vi "automated_Strain_attempt.vi"() -> ()   [LabVIEW 2014]
uses:
  <vilib>/vision/NI_Vision_Development_Module.lvlib
  <instrlib>/KD Scientific 2XX Series/KD Scientific 2XX Series.lvlib
panel:
  out "Diameter Selection":T1(plugin-control)
  out "di2":dbl
  out "di1":dbl
  out "d1":dbl
  out "d2":dbl
  out "Distances":dbl[](array[numeric])
  out "S2":dbl
  out "S1":dbl
  in  "Number of Cycles":i32
  in  "Min Pressure":dbl
  in  "Max Pressure":dbl
  out "Status":T2
  in  "stop 2":bool
  out "Delivered Volume":dbl
  out "Units":string
  in  "Baud Rate (9600)":u32(ring)=9600 items=["300"=300, "1200"=1200, "2400"=2400, "4800"=4800, "9600"=9600]
  in  "Withdrawal Settings":T3={"Flow Rate (5)"=5.0, "Volume (10)"=10.0, "Volume Units (ml)"=enum."milliliters (ml)", "Rate Units (ml/min.)"=enum."milliliters per minute (ml/min.)"} {"Volume (10)" format="%#.3g"}
  in  "Diameter (8.75 mm)":dbl=8.75
  in  "Infusion Settings":T3={"Flow Rate (5)"=5.0, "Volume (10)"=10.0, "Volume Units (ml)"=enum."milliliters (ml)", "Rate Units (ml/min.)"=enum."milliliters per minute (ml/min.)"}
  in  "Address (0)":i32 format="%0.0f"
  in  "error in (no error)":errorcluster
  in  "VISA resource name":refnum<visa-resource-name>="COM1"
  in  "stop 4":bool
  in  "stop":bool
  out "Strain Selection":T1(plugin-control)
  out "Particle Measurements (Pixels) (Particle Analysis 1)":dbl[][](array[numeric]) format="%.2f"
  out "subarray":dbl[](array[numeric])
  out "The diameter":dbl[](array[numeric])
  in  "stop (F)":bool
  out "Data from Transducer":dynamicdata(graph) caption="Voltage from Transducer V"
  out "Voltage from pressure transducer":dbl[](array[numeric])
  out "Pressure mm Hg":dbl[](graph)
  in  "Calibration factor":dbl[](array[numeric])
  in  "Zero Error":dbl[](array[numeric])
  out "pressure mm Hg":dbl[](array[numeric])
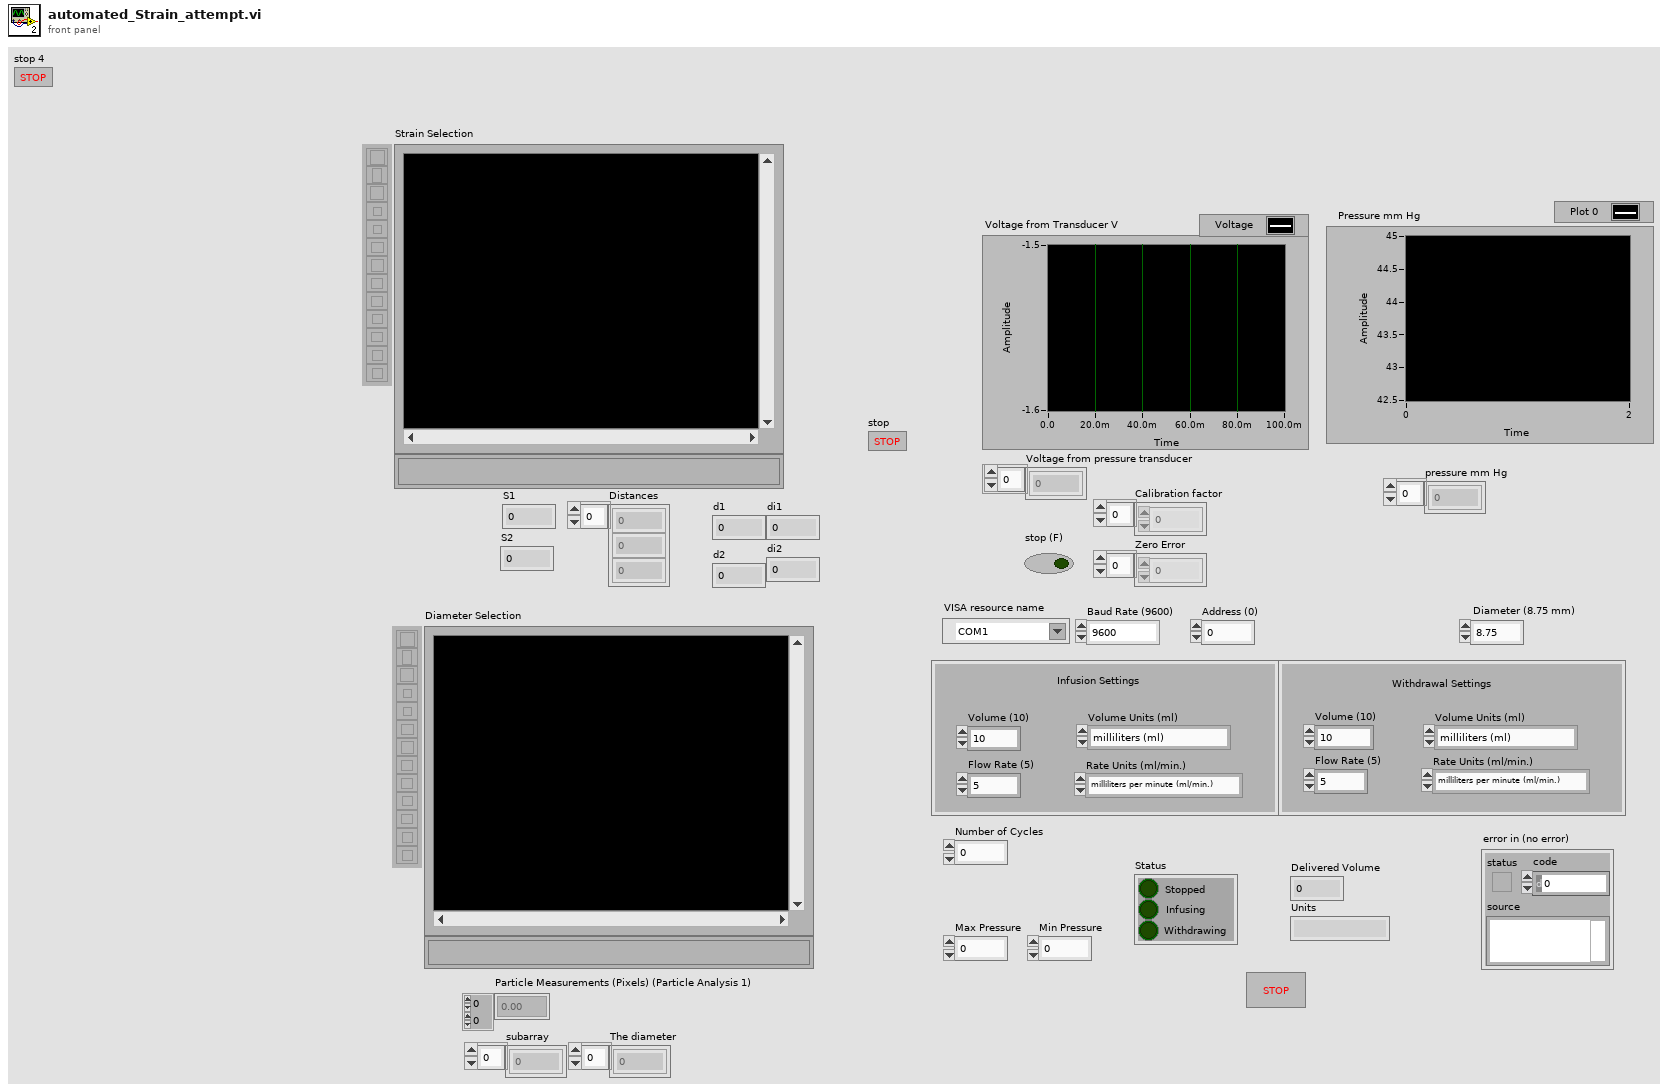
[diagram p1: front panel]
types:
  T1 = typedef "IMAQ Image.ctl" = refnum<image>
  T2 = cluster{"Stopped":bool, "Infusing":bool, "Withdrawing":bool}
  T3 = cluster{"Flow Rate (5)":dbl, "Volume (10)":dbl, "Volume Units (ml)":enum16{"milliliters (ml)", "microliters (ul)"}, "Rate Units (ml/min.)":enum16{"milliliters per minute (ml/min.)", "milliliters per hour (ml/hr.)", "microliters per minute (ul/min.)", "microliters per hour (ul/hr.)"}}
  T4 = typedef "Board Id" = u8
  T5 = typedef "ROI Descriptor" = cluster{"Global Rectangle":i32[], "Contours":cluster{"ID":enum32{"External", "Internal"}, "Type":u32, "Coordinates":i32[]}[]}
  T6 = enum16{"milliliters per minute (ml/min.)", "milliliters per hour (ml/hr.)", "microliters per minute (ul/min.)", "microliters per hour (ul/hr.)"}
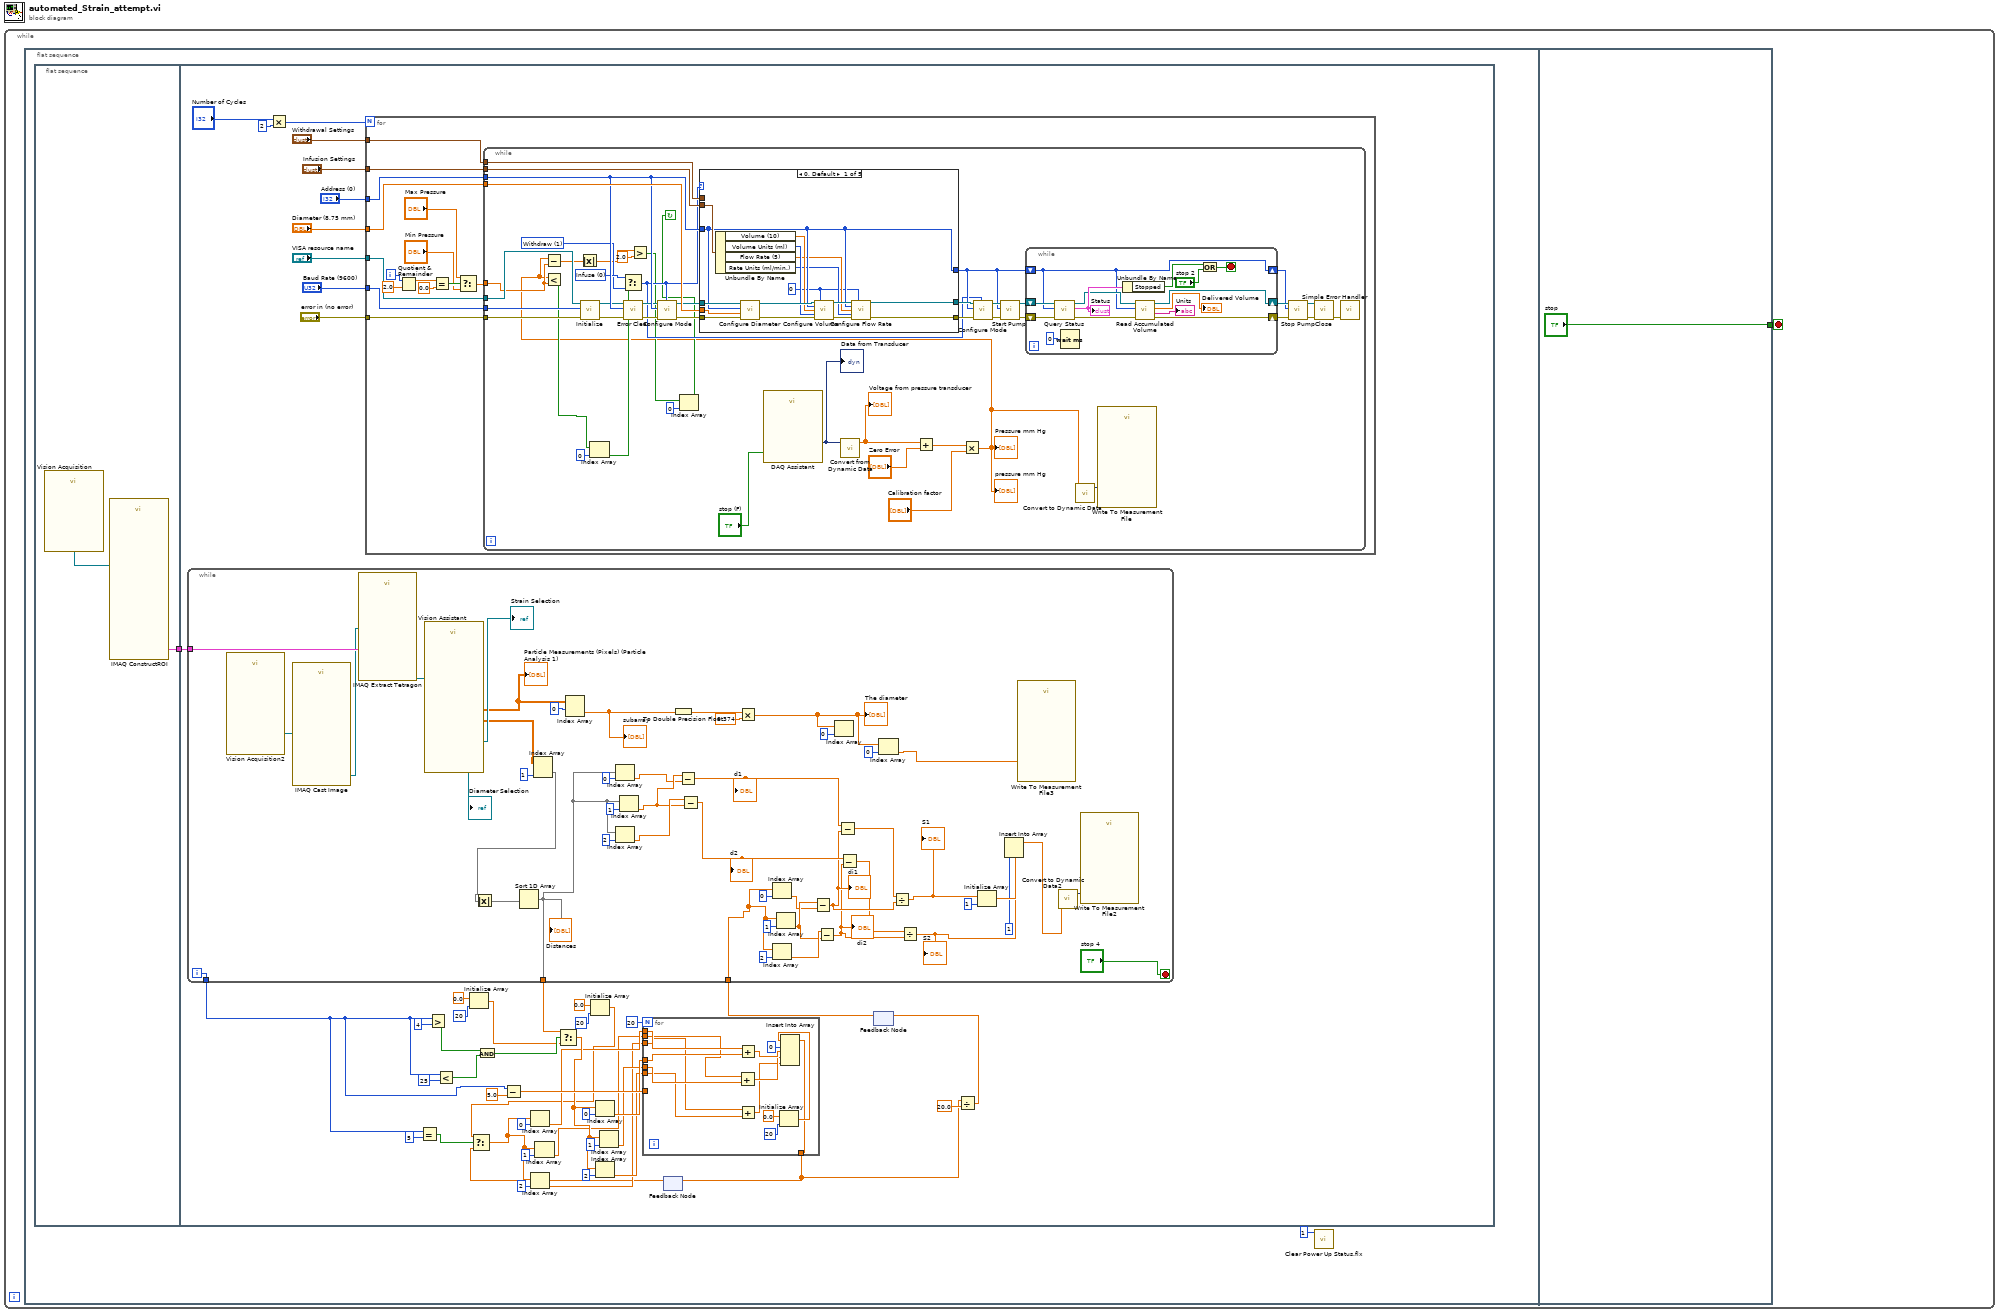
[diagram p0: block diagram]
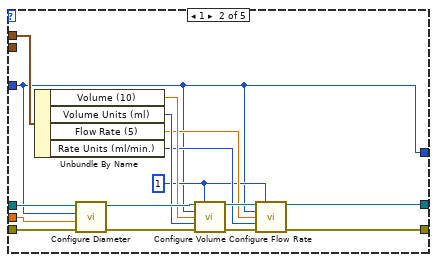
[diagram p2: hidden frame]
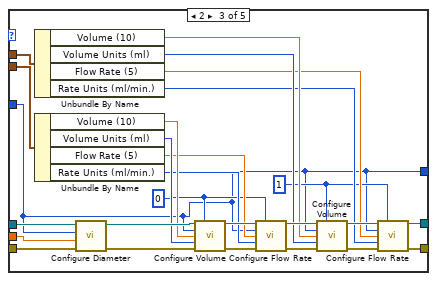
[diagram p3: hidden frame]
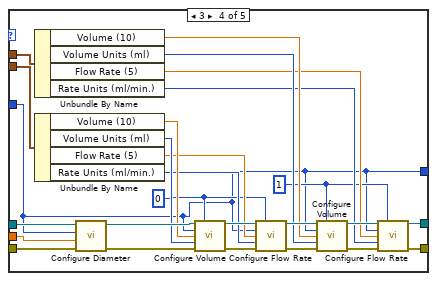
[diagram p4: hidden frame]
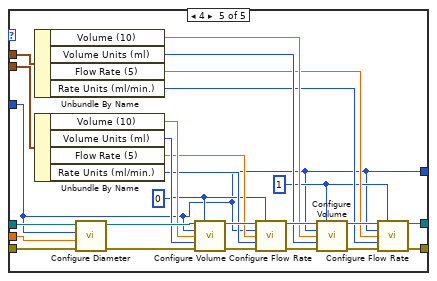
[diagram p5: hidden frame]
diagram:
  n1 = while {
    stop <- w1 stop-if-true
    n2 = flat-sequence {
      tunnel: ["stop"] -> w1
      frame #0 {
        n3 = flat-sequence {
          tunnel: [w4] -> w3
          tunnel: w3 -> [w53]
          frame #0 {
            n4 = call "Vision Acquisition"() -> ("Image Out"=w5:T1)  [unwired: 26 in, 1 out]
            n5 = call "IMAQ ConstructROI"("Image"=w5) -> ("ROI Descriptor Out"=w4:T5)  [unwired: 7 in, 3 out]
          }
          frame #1 {
            n6 = Multiply(x="Number of Cycles", y=2) -> (x*y=w52:i32)
            n7 = for {
              N: w52 -> [_]
              tunnel: "VISA resource name" -> [w82]
              tunnel: "error in (no error)" -> [w81]
              tunnel: "Infusion Settings" -> [w80]
              tunnel: "Withdrawal Settings" -> [w79]
              tunnel: "Diameter (8.75 mm)" -> [w78]
              tunnel: "Baud Rate (9600)" -> [w77]
              tunnel: "Address (0)" -> [w76]
              i -> [w74]
              n8 = Quotient & Remainder(x=w74, y=2.0) -> (x-y*floor(x/y)=w72:dbl)  [unwired: 1 out]
              n9 = Equal?(x=w72, y=0.0) -> (x = y?=w71:bool)
              n10 = Select(t="Max Pressure", s=w71, f="Min Pressure") -> (s? t:f=w68:dbl)
              n11 = while {
                tunnel: w82 -> [w129]
                tunnel: w81 -> [w128]
                tunnel: w80 -> [w127]
                tunnel: w79 -> [w126]
                tunnel: w78 -> [w125]
                tunnel: w77 -> [w124]
                tunnel: w76 -> [w123]
                tunnel: w68 -> [w100]
                stop <- w85 continue-if-true
                w102 = u16 1 items=["Withdraw"=1]
                w103 = u16 0 items=["Infuse"] ("Mode (infuse)")
                n12 = call <instrlib>:"Initialize.vi"("error in (no error)"=w128, "Baud Rate (9600)"=w124, "VISA resource name"=w129) -> ("error out"=w105:errorcluster, "VISA resource name out"=w104:refnum<visa-resource-name>)  [unwired: 7 in]
                n13 = call <instrlib>:"Error Clear.vi"("error in (no error)"=w105, "Address (0)"=w123, "VISA resource name"=w104) -> ("error out"=w106:errorcluster, "VISA resource name out"=w107:refnum<visa-resource-name>)  [unwired: 6 in, 1 out]
                n14 = call "DAQ Assistant"("stop (T)"="stop (F)") -> ("data"=w91:dynamicdata)  [unwired: 16 in, 2 out]
                "Data from Transducer" <- w91
                n15 = call "Convert from Dynamic Data"("Dynamic Data Type"=w91) -> ("Array"=w94:dbl[])  [unwired: 3 in]
                "Voltage from pressure transducer" <- w94
                n16 = Add(x=w94, y="Zero Error") -> (x+y=w92:dbl[])
                n17 = Multiply(x=w92, y="Calibration factor") -> (x*y=w84:dbl[])
                "Pressure mm Hg" <- w84
                "pressure mm Hg" <- w84
                n18 = Subtract(x=w84, y=w100) -> (x-y=w99:dbl[])
                n19 = Less?(x=w84, y=w100) -> (x < y?=w90:bool[])
                n20 = Absolute Value(x=w99) -> (abs(x)=w98:dbl[])
                n21 = Index Array(array=w90, index=0) -> (element=w88:bool)
                n22 = Select(t=w103, s=w88, f=w102) -> (s? t:f=w101:u16)
                n23 = Greater?(x=w98, y=2.0) -> (0:w87:bool[])
                n24 = call <instrlib>:"Configure Mode.vi"("Mode (infuse)"=w101, "error in (no error)"=w106, "Address (0)"=w123, "VISA resource name"=w107) -> ("error out"=w109:errorcluster, "VISA resource name out"=w108:refnum<visa-resource-name>)  [unwired: 6 in]
                n25 = Index Array(array=w87, index=0) -> (element=w85:bool)
                n26 = case shown="0, Default" w101 {
                  tunnel: w127 -> [w139 _ w187 w213 w239]
                  tunnel: w126 -> [_ w161 w186 w212 w238]
                  tunnel: w108 -> [w145 w160 w185 w211 w237]
                  tunnel: w109 -> [w144 w156 w184 w210 w236]
                  tunnel: w125 -> [w138 w152 w167 w193 w219]
                  tunnel: [w137 w146 w162 w188 w214] -> w110
                  tunnel: w123 -> [w137 w146 w162 w188 w214]
                  tunnel: [w132 w157 w164 w190 w216] -> w114
                  tunnel: [w131 w153 w163 w189 w215] -> w113
                  frame 0, Default {
                    w130 = 0
                    n27 = Unbundle By Name(w139) -> ("Volume (10)"=w136:dbl, "Volume Units (ml)"=w135:enum16{"milliliters (ml)", "microliters (ul)"}, "Flow Rate (5)"=w134:dbl, "Rate Units (ml/min.)"=w133:T6)
                    n28 = call <instrlib>:"Configure Diameter.vi"("error in (no error)"=w144, "Diameter (8.75 mm)"=w138, "Address (0)"=w137, "VISA resource name"=w145) -> ("error out"=w142:errorcluster, "VISA resource name out"=w143:refnum<visa-resource-name>)  [unwired: 6 in]
                    n29 = call <instrlib>:"Configure Volume.vi"("VISA resource name"=w143, "Mode (infuse)"=w130, "Address (0)"=w137, "Volume (100)"=w136, "Units (0: milliliters)"=w135, "error in (no error)"=w142) -> ("VISA resource name out"=w141:refnum<visa-resource-name>, "error out"=w140:errorcluster)  [unwired: 8 in]
                    n30 = call <instrlib>:"Configure Flow Rate.vi"("VISA resource name"=w141, "Mode (infuse)"=w130, "Address (0)"=w137, "Flow Rate (5)"=w134, "Units (0: milliliters per minute)"=w133, "error in (no error)"=w140) -> ("VISA resource name out"=w132:refnum<visa-resource-name>, "error out"=w131:errorcluster)  [unwired: 8 in]
                  }
                  frame 1 {
                    w147 = 1
                    n31 = Unbundle By Name(w161) -> ("Volume (10)"=w151:dbl, "Volume Units (ml)"=w150:enum16{"milliliters (ml)", "microliters (ul)"}, "Flow Rate (5)"=w149:dbl, "Rate Units (ml/min.)"=w148:T6)
                    n32 = call <instrlib>:"Configure Diameter.vi"("error in (no error)"=w156, "Diameter (8.75 mm)"=w152, "Address (0)"=w146, "VISA resource name"=w160) -> ("error out"=w155:errorcluster, "VISA resource name out"=w159:refnum<visa-resource-name>)  [unwired: 6 in]
                    n33 = call <instrlib>:"Configure Volume.vi"("VISA resource name"=w159, "Mode (infuse)"=w147, "Address (0)"=w146, "Volume (100)"=w151, "Units (0: milliliters)"=w150, "error in (no error)"=w155) -> ("VISA resource name out"=w158:refnum<visa-resource-name>, "error out"=w154:errorcluster)  [unwired: 8 in]
                    n34 = call <instrlib>:"Configure Flow Rate.vi"("VISA resource name"=w158, "Mode (infuse)"=w147, "Address (0)"=w146, "Flow Rate (5)"=w149, "Units (0: milliliters per minute)"=w148, "error in (no error)"=w154) -> ("VISA resource name out"=w157:refnum<visa-resource-name>, "error out"=w153:errorcluster)  [unwired: 8 in]
                  }
                  frame 2 {
                    w165 = 1
                    w166 = 0
                    n35 = Unbundle By Name(w186) -> ("Volume (10)"=w171:dbl, "Volume Units (ml)"=w170:enum16{"milliliters (ml)", "microliters (ul)"}, "Flow Rate (5)"=w169:dbl, "Rate Units (ml/min.)"=w168:T6)
                    n36 = Unbundle By Name(w187) -> ("Volume (10)"=w175:dbl, "Volume Units (ml)"=w174:enum16{"milliliters (ml)", "microliters (ul)"}, "Flow Rate (5)"=w173:dbl, "Rate Units (ml/min.)"=w172:T6)
                    n37 = call <instrlib>:"Configure Diameter.vi"("error in (no error)"=w184, "Diameter (8.75 mm)"=w167, "Address (0)"=w162, "VISA resource name"=w185) -> ("error out"=w179:errorcluster, "VISA resource name out"=w183:refnum<visa-resource-name>)  [unwired: 6 in]
                    n38 = call <instrlib>:"Configure Volume.vi"("VISA resource name"=w183, "Mode (infuse)"=w166, "Address (0)"=w162, "Volume (100)"=w175, "Units (0: milliliters)"=w174, "error in (no error)"=w179) -> ("VISA resource name out"=w182:refnum<visa-resource-name>, "error out"=w178:errorcluster)  [unwired: 8 in]
                    n39 = call <instrlib>:"Configure Flow Rate.vi"("VISA resource name"=w182, "Mode (infuse)"=w166, "Address (0)"=w162, "Flow Rate (5)"=w173, "Units (0: milliliters per minute)"=w172, "error in (no error)"=w178) -> ("VISA resource name out"=w181:refnum<visa-resource-name>, "error out"=w177:errorcluster)  [unwired: 8 in]
                    n40 = call <instrlib>:"Configure Volume.vi"("VISA resource name"=w181, "Mode (infuse)"=w165, "Address (0)"=w162, "Volume (100)"=w171, "Units (0: milliliters)"=w170, "error in (no error)"=w177) -> ("VISA resource name out"=w180:refnum<visa-resource-name>, "error out"=w176:errorcluster)  [unwired: 8 in]
                    n41 = call <instrlib>:"Configure Flow Rate.vi"("VISA resource name"=w180, "Mode (infuse)"=w165, "Address (0)"=w162, "Flow Rate (5)"=w169, "Units (0: milliliters per minute)"=w168, "error in (no error)"=w176) -> ("VISA resource name out"=w164:refnum<visa-resource-name>, "error out"=w163:errorcluster)  [unwired: 8 in]
                  }
                  frame 3 {
                    w191 = 1
                    w192 = 0
                    n42 = Unbundle By Name(w212) -> ("Volume (10)"=w197:dbl, "Volume Units (ml)"=w196:enum16{"milliliters (ml)", "microliters (ul)"}, "Flow Rate (5)"=w195:dbl, "Rate Units (ml/min.)"=w194:T6)
                    n43 = Unbundle By Name(w213) -> ("Volume (10)"=w201:dbl, "Volume Units (ml)"=w200:enum16{"milliliters (ml)", "microliters (ul)"}, "Flow Rate (5)"=w199:dbl, "Rate Units (ml/min.)"=w198:T6)
                    n44 = call <instrlib>:"Configure Diameter.vi"("error in (no error)"=w210, "Diameter (8.75 mm)"=w193, "Address (0)"=w188, "VISA resource name"=w211) -> ("error out"=w205:errorcluster, "VISA resource name out"=w209:refnum<visa-resource-name>)  [unwired: 6 in]
                    n45 = call <instrlib>:"Configure Volume.vi"("VISA resource name"=w209, "Mode (infuse)"=w192, "Address (0)"=w188, "Volume (100)"=w201, "Units (0: milliliters)"=w200, "error in (no error)"=w205) -> ("VISA resource name out"=w208:refnum<visa-resource-name>, "error out"=w204:errorcluster)  [unwired: 8 in]
                    n46 = call <instrlib>:"Configure Flow Rate.vi"("VISA resource name"=w208, "Mode (infuse)"=w192, "Address (0)"=w188, "Flow Rate (5)"=w199, "Units (0: milliliters per minute)"=w198, "error in (no error)"=w204) -> ("VISA resource name out"=w207:refnum<visa-resource-name>, "error out"=w203:errorcluster)  [unwired: 8 in]
                    n47 = call <instrlib>:"Configure Volume.vi"("VISA resource name"=w207, "Mode (infuse)"=w191, "Address (0)"=w188, "Volume (100)"=w197, "Units (0: milliliters)"=w196, "error in (no error)"=w203) -> ("VISA resource name out"=w206:refnum<visa-resource-name>, "error out"=w202:errorcluster)  [unwired: 8 in]
                    n48 = call <instrlib>:"Configure Flow Rate.vi"("VISA resource name"=w206, "Mode (infuse)"=w191, "Address (0)"=w188, "Flow Rate (5)"=w195, "Units (0: milliliters per minute)"=w194, "error in (no error)"=w202) -> ("VISA resource name out"=w190:refnum<visa-resource-name>, "error out"=w189:errorcluster)  [unwired: 8 in]
                  }
                  frame 4 {
                    w217 = 1
                    w218 = 0
                    n49 = Unbundle By Name(w238) -> ("Volume (10)"=w223:dbl, "Volume Units (ml)"=w222:enum16{"milliliters (ml)", "microliters (ul)"}, "Flow Rate (5)"=w221:dbl, "Rate Units (ml/min.)"=w220:T6)
                    n50 = Unbundle By Name(w239) -> ("Volume (10)"=w227:dbl, "Volume Units (ml)"=w226:enum16{"milliliters (ml)", "microliters (ul)"}, "Flow Rate (5)"=w225:dbl, "Rate Units (ml/min.)"=w224:T6)
                    n51 = call <instrlib>:"Configure Diameter.vi"("error in (no error)"=w236, "Diameter (8.75 mm)"=w219, "Address (0)"=w214, "VISA resource name"=w237) -> ("error out"=w231:errorcluster, "VISA resource name out"=w235:refnum<visa-resource-name>)  [unwired: 6 in]
                    n52 = call <instrlib>:"Configure Volume.vi"("VISA resource name"=w235, "Mode (infuse)"=w218, "Address (0)"=w214, "Volume (100)"=w227, "Units (0: milliliters)"=w226, "error in (no error)"=w231) -> ("VISA resource name out"=w234:refnum<visa-resource-name>, "error out"=w230:errorcluster)  [unwired: 8 in]
                    n53 = call <instrlib>:"Configure Flow Rate.vi"("VISA resource name"=w234, "Mode (infuse)"=w218, "Address (0)"=w214, "Flow Rate (5)"=w225, "Units (0: milliliters per minute)"=w224, "error in (no error)"=w230) -> ("VISA resource name out"=w233:refnum<visa-resource-name>, "error out"=w229:errorcluster)  [unwired: 8 in]
                    n54 = call <instrlib>:"Configure Volume.vi"("VISA resource name"=w233, "Mode (infuse)"=w217, "Address (0)"=w214, "Volume (100)"=w223, "Units (0: milliliters)"=w222, "error in (no error)"=w229) -> ("VISA resource name out"=w232:refnum<visa-resource-name>, "error out"=w228:errorcluster)  [unwired: 8 in]
                    n55 = call <instrlib>:"Configure Flow Rate.vi"("VISA resource name"=w232, "Mode (infuse)"=w217, "Address (0)"=w214, "Flow Rate (5)"=w221, "Units (0: milliliters per minute)"=w220, "error in (no error)"=w228) -> ("VISA resource name out"=w216:refnum<visa-resource-name>, "error out"=w215:errorcluster)  [unwired: 8 in]
                  }
                }
                n56 = call <instrlib>:"Configure Mode.vi"("Mode (infuse)"=w101, "error in (no error)"=w113, "Address (0)"=w110, "VISA resource name"=w114) -> ("error out"=w111:errorcluster, "VISA resource name out"=w112:refnum<visa-resource-name>)  [unwired: 6 in]
                n57 = call <instrlib>:"Start Pump.vi"("error in (no error)"=w111, "Address (0)"=w110, "VISA resource name"=w112) -> ("error out"=w121:errorcluster, "VISA resource name out"=w122:refnum<visa-resource-name>)  [unwired: 7 in]
                n58 = while {
                  shift-right: [w242] -> w118
                  shift-left: w110 -> [w242]
                  shift-right: [w244] -> w120
                  shift-left: w122 -> [w250]
                  shift-right: [w243] -> w119
                  shift-left: w121 -> [w251]
                  stop <- w248 stop-if-true
                  n59 = call <instrlib>:"Query Status.vi"("error in (no error)"=w251, "Address (0)"=w242, "VISA resource name"=w250) -> ("error out"=w253:errorcluster, "Status"=w249:T2, "VISA resource name out"=w245:refnum<visa-resource-name>)  [unwired: 6 in]
                  "Status" <- w249
                  n60 = Wait (ms)(milliseconds to wait=u32 0) -> ()  [unwired: 1 out]
                  n61 = Unbundle By Name(w249) -> ("Stopped"=w247:bool)
                  n62 = call <instrlib>:"Read Accumulated Volume.vi"("error in (no error)"=w253, "Address (0)"=w242, "VISA resource name"=w245) -> ("error out"=w243:errorcluster, "Units"=→"Units":string, "Delivered Volume"=→"Delivered Volume":dbl, "VISA resource name out"=w244:refnum<visa-resource-name>)  [unwired: 5 in]
                  n63 = Or(x=w247, y="stop 2") -> (x .or. y?=w248:bool)
                }
                n64 = call "Convert to Dynamic Data"("Array"=w84) -> ("Dynamic Data Type"=w83:dynamicdata)  [unwired: 3 in]
                n65 = call "Write To Measurement File"("Signals"=w83) -> ()  [unwired: 16 in, 3 out]
                n66 = call <instrlib>:"Stop Pump.vi"("error in (no error)"=w119, "Address (0)"=w118, "VISA resource name"=w120) -> ("error out"=w116:errorcluster, "VISA resource name out"=w115:refnum<visa-resource-name>)  [unwired: 7 in]
                n67 = call <instrlib>:"Close.vi"("error in (no error)"=w116, "VISA resource name"=w115) -> ("error out"=w117:errorcluster)  [unwired: 9 in]
                n68 = call <vilib>:"Simple Error Handler.vi"("error in (no error)"=w117) -> ()  [unwired: 4 in, 5 out]
              }
            }
            n69 = Initialize Array(0.0 ("element"), 20 ("dimension size")) -> (w6:dbl[])
            n70 = Initialize Array(0.0 ("element"), 20 ("dimension size")) -> (w15:dbl[])
            n71 = feedback #1() -> (w13:dbl[])  [unwired: 1 in]
            n72 = feedback #2() -> (w9:dbl[])  [unwired: 1 in]
            n73 = while {
              tunnel: w53 -> [w301]
              tunnel: [w256] -> w18
              tunnel: [w255] -> w35
              tunnel: w9 -> [w254]
              i -> [w256]
              stop <- "stop 4" stop-if-true
              n74 = call "Vision Acquisition2"() -> ("Image Out"=w291:T1)  [unwired: 25 in, 2 out]
              n75 = call "IMAQ Cast Image"("Image Src"=w291) -> ("Image Dst Out"=w298:T1)  [unwired: 9 in, 1 out]
              n76 = call-poly "IMAQ Extract Tetragon"("ROI Descriptor"=w301, "Image Src"=w298) -> ("Image Dst Out"=w299:T1)  [unwired: 8 in, 1 out]
              n77 = call "Vision Assistant"("Image In"=w299) -> ("Image Out"=→"Strain Selection":T1, "Particle Measurements (Pixels) (Particle Analysis 1)"=w297:dbl[][], "Particle Measurements (Pixels) (Particle Analysis 2)"=w286:dbl[][], "Image Buffer (Image Buffer 4)"=→"Diameter Selection":T1)  [unwired: 20 in, 3 out]
              "Particle Measurements (Pixels) (Particle Analysis 1)" <- w297
              n78 = Index Array(array=w286, index (col)=1 ("disabled index (col)")) -> (element=w279:dbl[])  [unwired: 1 in]
              n79 = Absolute Value(x=w279) -> (abs(x)=w278:dbl[])
              n80 = Sort 1D Array(array=w278) -> (sorted array=w255:dbl[])
              "Distances" <- w255
              n81 = Index Array(array=w297, index (row)=0) -> (element=w295:dbl[])  [unwired: 1 in]
              "subarray" <- w295
              n82 = Index Array(array=w255, index=0) -> (element=w261:dbl)
              n83 = Index Array(array=w255, index=2) -> (element=w263:dbl)
              n84 = Index Array(array=w255, index=1) -> (element=w262:dbl)
              n85 = To Double Precision Float(number=w295) -> (double precision float=w294:dbl[])
              n86 = Subtract(x=w262, y=w261) -> (x-y=w274:dbl)
              "d1" <- w274
              n87 = Subtract(x=w263, y=w262) -> (x-y=w273:dbl)
              "d2" <- w273
              n88 = Multiply(x=w294, y=0.374) -> (x*y=w288:dbl[])
              "The diameter" <- w288
              n89 = Index Array(array=w254, index=0) -> (element=w258:dbl)
              n90 = Index Array(array=w254, index=2) -> (element=w260:dbl)
              n91 = Index Array(array=w254, index=1) -> (element=w259:dbl)
              n92 = Subtract(x=w259, y=w258) -> (x-y=w271:dbl)
              "di1" <- w271
              n93 = Subtract(x=w260, y=w259) -> (x-y=w269:dbl)
              "di2" <- w269
              n94 = Index Array(array=w288, index=0) -> ()  [unwired: 1 out]
              n95 = Subtract(x=w274, y=w271) -> (x-y=w272:dbl)
              n96 = Subtract(x=w273, y=w269) -> (x-y=w270:dbl)
              n97 = Index Array(array=w288, index=0) -> (element=w287:dbl)
              n98 = Divide(x=w272, y=w271) -> (x/y=w268:dbl)
              "S1" <- w268
              n99 = Divide(x=w270, y=w269) -> (x/y=w267:dbl)
              "S2" <- w267
              n100 = Initialize Array(w268, 1 ("dimension size")) -> (w281:dbl[])
              n101 = Insert Into Array(array=w281, index=1, new element=w267) -> (w266:dbl[])
              n102 = call "Write To Measurement File3"("Signals"=w287) -> ()  [unwired: 16 in, 3 out]
              n103 = call "Convert to Dynamic Data2"("Array"=w266) -> ("Dynamic Data Type"=w265:dynamicdata)  [unwired: 3 in]
              n104 = call "Write To Measurement File2"("Signals"=w265) -> ()  [unwired: 16 in, 3 out]
            }
            n105 = Equal?(x=w18, y=5) -> (x = y?=w16:bool)
            n106 = Greater?(x=w18, y=4) -> (0:w42:bool)
            n107 = Less?(x=w18, y=25) -> (x < y?=w41:bool)
            n108 = Select(t=w15, s=w16, f=w13) -> (s? t:f=w14:dbl[])
            n109 = And(x=w42, y=w41) -> (x .and. y?=w36:bool)
            n110 = Subtract(x=w18, y=5.0) -> (x-y=w34:dbl)
            n111 = Index Array(array=w14, index=0) -> (element=w21:dbl)
            n112 = Index Array(array=w14, index=2) -> (element=w19:dbl)
            n113 = Index Array(array=w14, index=1) -> (element=w20:dbl)
            n114 = Select(t=w35, s=w36, f=w6) -> (s? t:f=w28:dbl[])
            n115 = Index Array(array=w28, index=0) -> (element=w27:dbl)
            n116 = Index Array(array=w28, index=2) -> (element=w25:dbl)
            n117 = Index Array(array=w28, index=1) -> (element=w26:dbl)
            n118 = for {
              N: 20 -> [_]
              tunnel: w34 -> [_]
              tunnel: w27 -> [w67]
              tunnel: w26 -> [w65]
              tunnel: w25 -> [w63]
              tunnel: w21 -> [w66]
              tunnel: w20 -> [w64]
              tunnel: w19 -> [w62]
              tunnel: [w54] -> w11
              n119 = Add(x=w64, y=w65) -> (x+y=w56:dbl)
              n120 = Add(x=w66, y=w67) -> (x+y=w57:dbl)
              n121 = Add(x=w62, y=w63) -> (x+y=w55:dbl)
              n122 = Initialize Array(0.0 ("element"), 20 ("dimension size")) -> (w58:dbl[])
              n123 = Insert Into Array(array=w58, index=0, new element #1=w57, new element #2=w56, new element #3=w55) -> (w54:dbl[])
            }
            n124 = feedback-in #1(w11) -> ()
            n125 = Divide(x=w11, y=20.0) -> (x/y=w10:dbl[])
            n126 = feedback-in #2(w10) -> ()
          }
        }
        n127 = call <vilib>:"Clear Power Up Status.flx"("Board ID"=T4 1) -> ()  [unwired: 6 in, 2 out]
      }
      frame #1 {
      }
    }
  }
